vi "Set Angle Speed.vi"(11 "Axes":T1) -> (3 "Angle Speed":dbl)   [LabVIEW 2011]
uses:
  Robot Global Data.vi
panel:
  in  "Angle Motor Scaling":dbl(slide)=0.4 scale=0.0..1.0
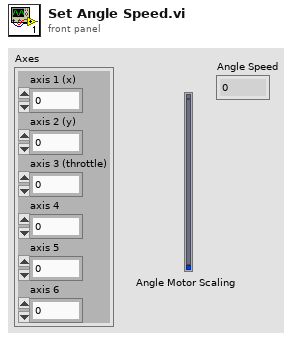
[diagram p1: front panel]
types:
  T1 = cluster{"axis 1 (x)":dbl, "axis 2 (y)":dbl, "axis 3 (throttle)":dbl, "axis 4":dbl, "axis 5":dbl, "axis 6":dbl}
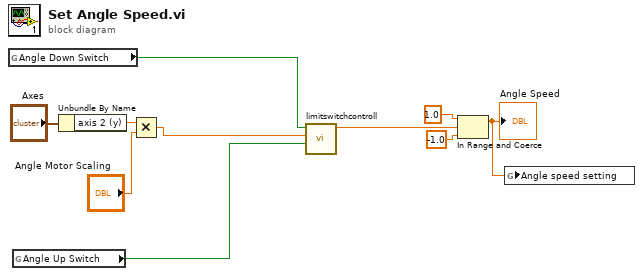
[diagram p0: block diagram]
diagram:
  n1 = global read "Robot Global Data.vi" "Angle Down Switch"() -> (w3:bool)
  n2 = global read "Robot Global Data.vi" "Angle Up Switch"() -> (w4:bool)
  n3 = Unbundle By Name("Axes") -> ("axis 2 (y)"=w7:dbl)
  n4 = Multiply(x=w7, y="Angle Motor Scaling") -> (x*y=w2:dbl)
  n5 = call "limitswitchcontroll.vi"("Up Switch"=w4, "Numeric"=w2, "Down Switch"=w3) -> ("t"=w1:dbl)  [unwired: 8 in]
  n6 = In Range and Coerce(upper limit=1.0, x=w1, lower limit=-1.0) -> (coerced(x)=w5:dbl)  [unwired: 1 out]
  "Angle Speed" <- w5
  n7 = global write "Robot Global Data.vi" "Angle speed setting"(w5) -> ()
